vi "DMM DCVM TTL0 PXI HW Trigger Delay.vi"() -> ()   [LabVIEW 2021]
uses:
  DMM_DC-RMS Voltage Measurement/Typedefs/Function Settings.ctl
  <instrlib>/niDMM/nidmm.llb/niDMM Resolution in Digits.ctl
  DMM_DC-RMS Voltage Measurement/Typedefs/Timing & Trigger Settings.ctl
  <instrlib>/niDMM/nidmm.llb/niDMM Trigger.ctl
  <instrlib>/niDMM/nidmm.llb/niDMM Slope.ctl
  DMM_DC-RMS Voltage Measurement/Typedefs/Measurement.ctl
  DMM Mixed Measurements/DMM Mixed Meas Typedefs/DMM Execution Settings.ctl
  Signal Voltage Generation/Typedefs/Signal Generation Settings.ctl
  Signal Voltage Generation/Typedefs/Generation Types.ctl
  Signal Voltage Generation/Typedefs/Single Tone Settings.ctl
  Signal Voltage Generation/Typedefs/Waveform Type.ctl
  Signal Voltage Generation/Typedefs/Tone Settings.ctl
  Synchronization/Typedefs/Routing Path.ctl
  Synchronization/Typedefs/Routing Signal.ctl
  DMM_DC-RMS Voltage Measurement/DMM_DC-RMS Voltage Measurement.lvlib
  Signal Voltage Generation/DAQ_Signal Voltage Generation.lvlib
  Synchronization/DAQ_Synchronization.lvlib
  DMM Mixed Measurements/DMM_Mixed Measurement.lvlib
panel:
  in  "Routing paths":T1[](array[typedef])=[{"Signal"=enum."Start Trigger", "Output Terminal"="/DAQ_6361/PXI_Trig0"}]
  out "error out 2":errorcluster caption="error out"
  in  "Signal Generation Settings":T3={"Generation Type"=enum."Single Tone", "Generation Time (s)"=4.0, "Voltage Offset (v)"=0.0, "Single Tone Settings"={"Waveform Type"=enum."Sine Wave", "Frequency (Hz)"=100.0, "Amplitude (V)"=1.0, "Duty Cycle (%)"=50.0}, "Multi Tone Settings"=[]} {"Voltage Offset (v)" format="%.2p"; "Generation Time (s)" format="%.2p"; "Multi Tone Settings"."Amplitude (V)" format="%.2p"; "Multi Tone Settings"."Frequency (Hz)" format="%.2p"; "Single Tone Settings"."Duty Cycle (%)" format="%.2p"; "Single Tone Settings"."Amplitude (V)" format="%.2p"; "Single Tone Settings"."Frequency (Hz)" format="%.2p"}
  out "error out":errorcluster
  out "DMM Execution Settings":T8={"Absolute\nResolution"=2.4999999999999998e-05, "Input Resistance\n(Ohm)"=1000000.0, "Digits\nResolution"=5.5, "Range"=5.0, "Minimum\nFrequency (Hz)"=40.0, "Aperture\nTime (s)"=0.1, "Auto Range\nValue"=5.0, "Settle\nTime (s)"=1.0, "Function"=2} {"Function" items=["DC Volts"=1, "AC Volts"=2, "DC Current"=3, "AC Current"=4, "2-Wire Resistance"=5, "4-Wire Resistance"=101, "Frequency"=104, "Period"=105, "AC Volts DC Coupled"=1001, "Diode"=1002, "Waveform Voltage"=1003, "Waveform Current"=1004, "Capacitance"=1005, "Inductance"=1006, "Temperature"=108]; "Absolute\nResolution" format="%#_6p"; "Input Resistance\n(Ohm)" format="%#_6p"; "Range" format="%#_6p"; "Minimum\nFrequency (Hz)" format="%#_6p"; "Aperture\nTime (s)" format="%#_6p"; "Auto Range\nValue" format="%#_6p"; "Settle\nTime (s)" format="%#_6p"}
  out "Measurement":T9={"Measured Value"=0.7067717942826807, "Out of Range"=FALSE, "Unit"="V (ac)", "Measurement"="706.772mV (ac)"} {"Measured Value" format="%^#_9e"}
  in  "Timing and Trigger Settings":T10={"AC Min Frequency (Hz)"=40.0, "Aperture Time (s)"=-1.0, "Settle Time (s)"=-1.0, "Trigger Settings"={"Trigger Delay (sec)"=1.0, "Enable Trigger?"=TRUE, "Trigger Source"=enum."TTL 0", "Slope"=enum."Rising Edge"}} {"Trigger Settings"."Trigger Delay (sec)" format="%.4f"; "AC Min Frequency (Hz)" format="%.2f"}
  in  "Function Settings":T13={"Range and Function"=enum."AC 2 V", "Resolution in Digits"=5.5} {"Resolution in Digits" items=["3 1/2"=3.5, "4 1/2"=4.5, "5 1/2"=5.5, "6 1/2"=6.5, "7 1/2"=7.5]}
  in  "DMM Resource Name":refnum<k15>="DMM_4080"
  # "Frequency (Hz)"
  # "Amplitude (V)"
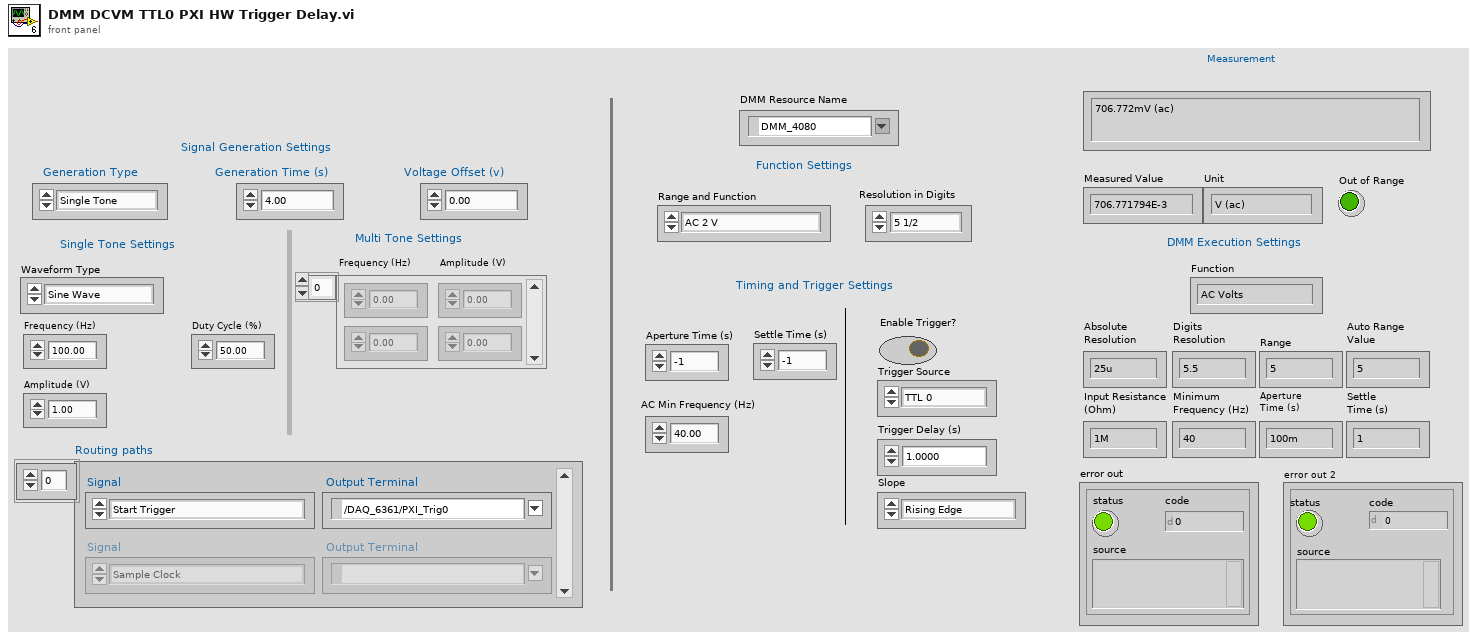
[diagram p1: front panel]
types:
  T1 = typedef "DAQ_Synchronization.lvlib/Routing Path.ctl" = cluster{"Signal":T2, "Output Terminal":tag}
  T2 = typedef "DAQ_Synchronization.lvlib/Routing Signal.ctl" = enum16{"Sample Clock", "Start Trigger"}
  T3 = typedef "DAQ_Signal Voltage Generation.lvlib/Signal Generation Settings.ctl" = cluster{"Generation Type":T4, "Generation Time (s)":dbl, "Voltage Offset (v)":dbl, "Single Tone Settings":T5, "Multi Tone Settings":T7[]}
  T4 = typedef "DAQ_Signal Voltage Generation.lvlib/Generation Types.ctl" = enum16{"Single Tone", "Multi Tone"}
  T5 = typedef "DAQ_Signal Voltage Generation.lvlib/Single Tone Settings.ctl" = cluster{"Waveform Type":T6, "Frequency (Hz)":dbl, "Amplitude (V)":dbl, "Duty Cycle (%)":dbl}
  T6 = typedef "DAQ_Signal Voltage Generation.lvlib/Waveform Type.ctl" = enum16{"Sine Wave", "Square Wave"}
  T7 = typedef "DAQ_Signal Voltage Generation.lvlib/Tone Settings.ctl" = cluster{"Frequency (Hz)":dbl, "Amplitude (V)":dbl}
  T8 = typedef "DMM_Mixed Measurement.lvlib/DMM Execution Settings.ctl" = cluster{"Absolute\nResolution":dbl, "Input Resistance\n(Ohm)":dbl, "Digits\nResolution":dbl, "Range":dbl, "Minimum\nFrequency (Hz)":dbl, "Aperture\nTime (s)":dbl, "Auto Range\nValue":dbl, "Settle\nTime (s)":dbl, "Function":i32}
  T9 = typedef "DMM_DC-RMS Voltage Measurement.lvlib/Measurement.ctl" = cluster{"Measured Value":dbl, "Out of Range":bool, "Unit":string, "Measurement":string}
  T10 = typedef "DMM_DC-RMS Voltage Measurement.lvlib/Timing & Trigger Settings.ctl" = cluster{"AC Min Frequency (Hz)":dbl, "Aperture Time (s)":dbl, "Settle Time (s)":dbl, "Trigger Settings":cluster{"Trigger Delay (sec)":dbl, "Enable Trigger?":bool, "Trigger Source":T11, "Slope":T12}}
  T11 = typedef "niDMM Trigger.ctl" = enum16{"Immediate", "External", "TTL 0", "TTL 1", "TTL 2", "TTL 3", "TTL 4", "TTL 5", "TTL 6", "Software", "TTL 7", "PXI Star", "LBR Trig 1", "Aux Trig 1"}
  T12 = typedef "niDMM Slope.ctl" = enum16{"Rising Edge", "Falling Edge"}
  T13 = typedef "DMM_DC-RMS Voltage Measurement.lvlib/Function Settings.ctl" = cluster{"Range and Function":enum16{"DC Voltage Auto Range", "DC 100 mV", "DC 1 V ", "DC 10 V", "DC 100 V", "DC 300 V", " ", "AC Voltage Auto Range", "AC 50 mV", "AC 200 mV", "AC 500 mV", "AC 2 V", "AC 5 V", "AC 20 V", "AC 50 V", "AC 300 V"}, "Resolution in Digits":T14}
  T14 = typedef "niDMM Resolution in Digits.ctl" = dbl
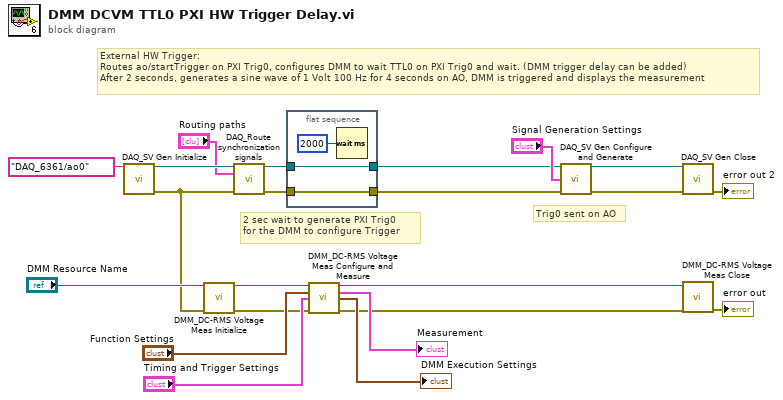
[diagram p0: block diagram]
diagram:
  # "Trig0 sent on AO"
  # "2 sec wait to generate PXI Trig0\nfor the DMM to configure Trigger"
  # "External HW Trigger: \nRoutes ao/startTrigger on PXI Trig0, configures DMM to wait TTL0 on PXI Trig0 and wait. (DMM trigger delay can be added)\nAfter 2 seconds, generates a sine wave of 1 Volt 100 Hz for 4 seconds on AO, DMM is triggered and displays the measurement"
  n1 = call "DAQ_SV Gen Initialize.vi"("Physical Channels"=tag "DAQ_6361/ao0") -> ("DAQmx Task Out"=w14:refnum<k21>, "error out"=w13:errorcluster)  [unwired: 13 in]
  n2 = call "DMM_DC-RMS Voltage Meas Initialize.vi"("DMM Resource Name"="DMM Resource Name", "error in"=w13) -> ("DMM Handle Out"=w10:refnum<k15>, "error out"=w9:errorcluster)  [unwired: 12 in]
  n3 = call "DAQ_Route synchronization signals.vi"("DAQmx Task In"=w14, "Routing paths"="Routing paths", "error in"=w13) -> ("DAQmx Task Out"=w5:refnum<k21>, "error out"=w4:errorcluster)  [unwired: 11 in]
  n4 = flat-sequence {
    tunnel: w5 -> [w25]
    tunnel: w4 -> [w24]
    tunnel: [w25] -> w3
    tunnel: [w24] -> w2
    frame #0 {
      n5 = Wait (ms)(milliseconds to wait=u32 2000) -> ()  [unwired: 1 out]
    }
  }
  n6 = call "DMM_DC-RMS Voltage Meas Configure and Measure.vi"("DMM Handle In"=w10, "Function Settings"="Function Settings", "Timing and Trigger Settings"="Timing and Trigger Settings", "error in"=w9) -> ("DMM Handle Out"=w19:refnum<k15>, "Measurement"=→"Measurement":T9, "DMM Execution Settings"=→"DMM Execution Settings":T8, "error out"=w8:errorcluster)  [unwired: 8 in]
  n7 = call "DAQ_SV Gen Configure and Generate.vi"("DAQmx Task In"=w3, "Signal Generation Settings"="Signal Generation Settings", "error in"=w2) -> ("DAQmx Task Out"=w22:refnum<k21>, "error out"=w6:errorcluster)  [unwired: 10 in, 1 out]
  n8 = call "DAQ_SV Gen Close.vi"("DAQmx Task In"=w22, "error in"=w6) -> ("error out"=→"error out 2":errorcluster)  [unwired: 13 in]
  n9 = call "DMM_DC-RMS Voltage Meas Close.vi"("DMM Handle In"=w19, "error in"=w8) -> ("error out"=→"error out":errorcluster)  [unwired: 13 in]
